vi "PyrometerSettings.vi"() -> ()   [LabVIEW 2018]
uses:
  C:/Users/bowenm/Git/Acquisition/Instruments/ImagingPyrometer/Kineses/ThorLabs.MotionControl.KCube.DCServoCLI.dll
  Kineses/ThorLabs.MotionControl.KCube.DCServoCLI.dll
  Global Variables.vi
  <vilib>/Utility/file.llb/Read Delimited Spreadsheet (string).vi
  C:/Users/bowenm/Git/Acquisition/Instruments/ImagingPyrometer/Kineses/Thorlabs.MotionControl.Controls.dll
  Kineses/Thorlabs.MotionControl.Controls.dll
  <instrlib>/Thorlabs_FW102C/Thorlabs_FW102C.lvlib
panel:
  in  "Set":bool
  out "Position Error":bool
  out "tdms file out":refnum<k34>
  out "RFW wls":string[](array[string])=["800", "900", "850", "750", "700", "600"]
  out "TFW wls":string[](array[string])=["1000", "850", "800", "700", "650", "600"]
  in  "Tab Control":enum32{"400-700nm", "700-1100nm"}(tab)
  in  "VisTFW Wavelength":u16(ring) caption="Wavelength 1" items=["600", "650", "700"]
  in  "VisRFW Wavelength":u16(ring) caption="Wavelength 2" items=["600", "700"]
  in  "NIRRFW Wavelengths":u16(ring) caption="Wavelength 2" items=["700", "750", "800", "850", "900"]
  in  "NIRTFW Wavelengths":u16(ring) caption="Wavelength 1" items=["700", "800", "850", "1000"]
  out "NDFs":dbl[](array[numeric])=[0.0, 20.0, 40.0, 60.0, 80.0, 100.0]
  in  "NeutralDensityFilter":u16(ring) items=["0", "20", "40", "60", "80", "100"]
  in  "NDFW Serial Port":string="COM17"
  out "NDFW102C out":i32
  out "RFW102C out":i32=1
  in  "RFW Serial Port":string="COM3"
  out "error out":errorcluster
  out "TFW102C out":i32
  in  "TFW Serial Port":string="COM4"
  out "MotorMoving":bool
  out "Device":refnum<k24>
  in  "stop":bool
  in  "KCubeDCServoControl":refnum<k24>(container)
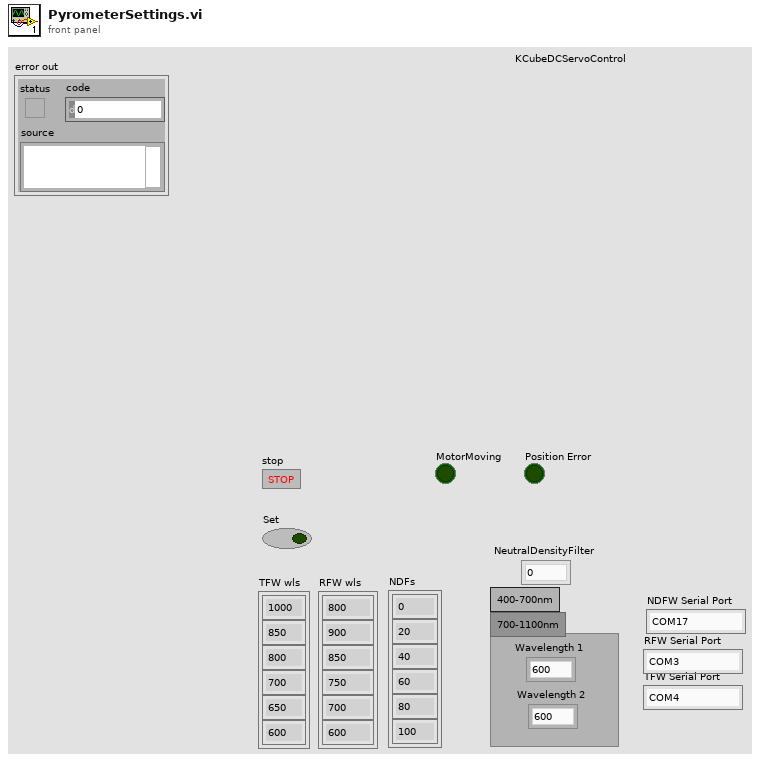
[diagram p1: front panel]
types:
  T1 = enum16{"open", "open or create", "create or replace", "create", "open (read-only)"}
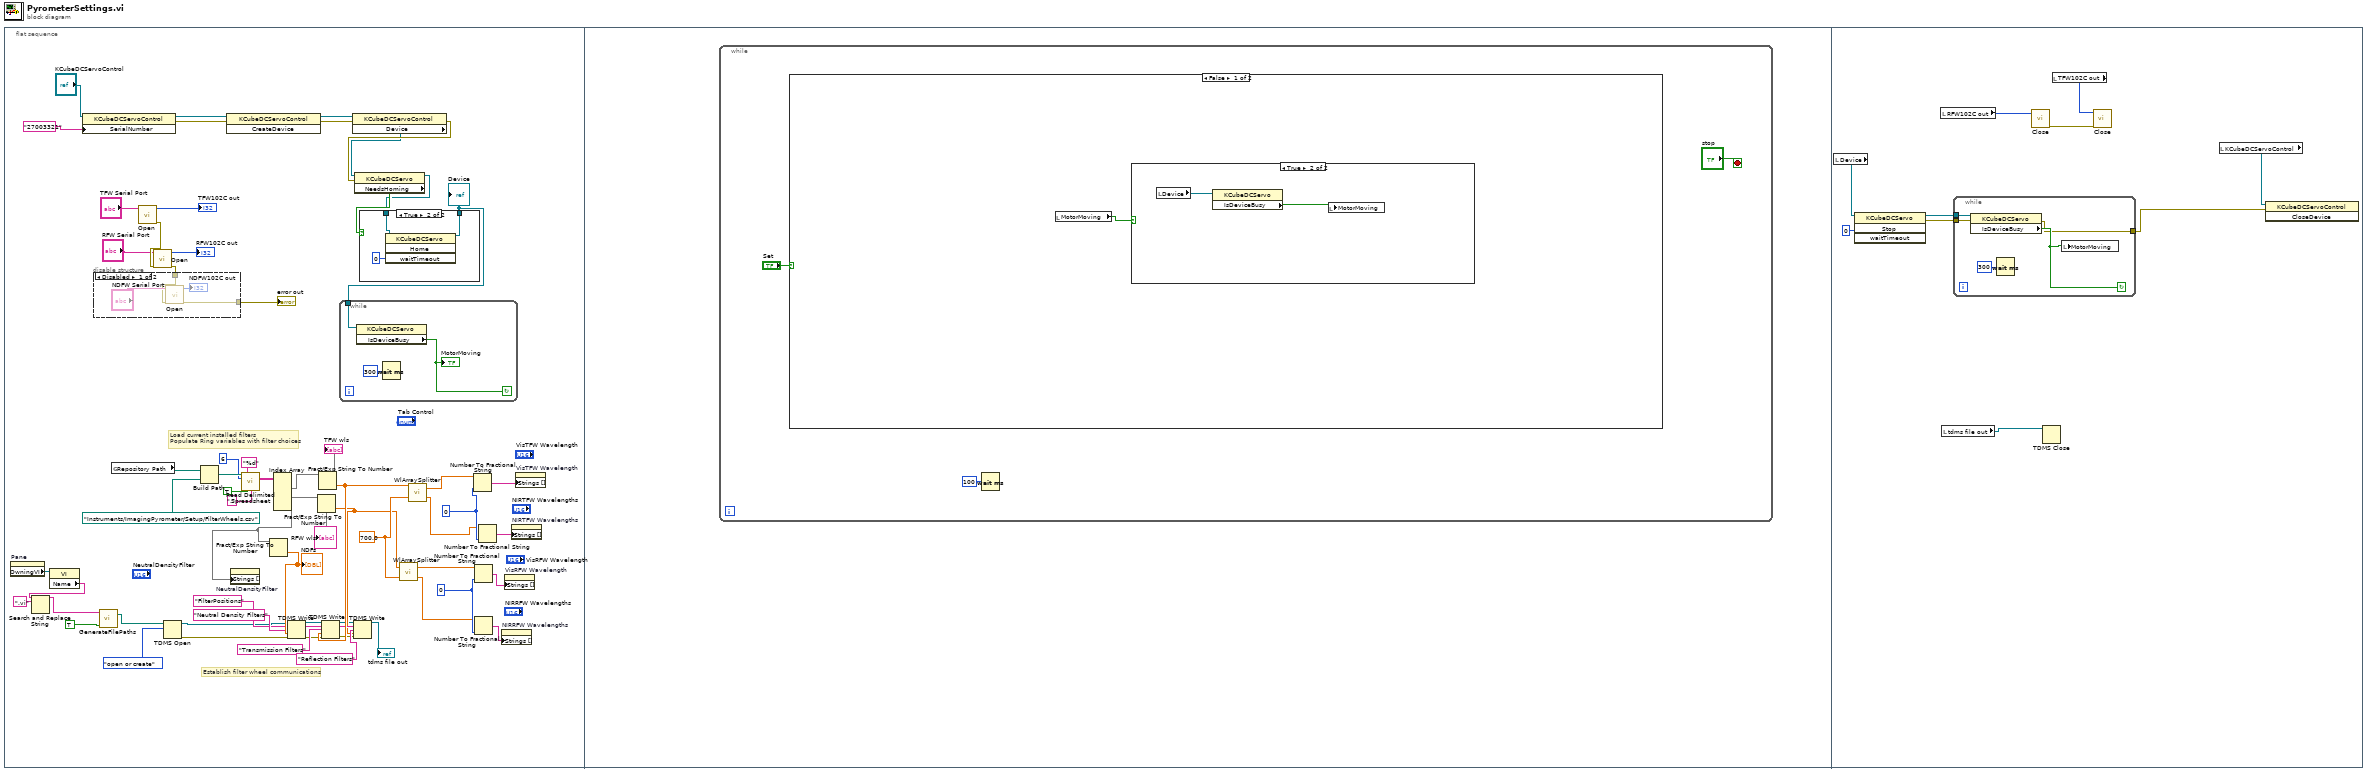
[diagram p0: block diagram]
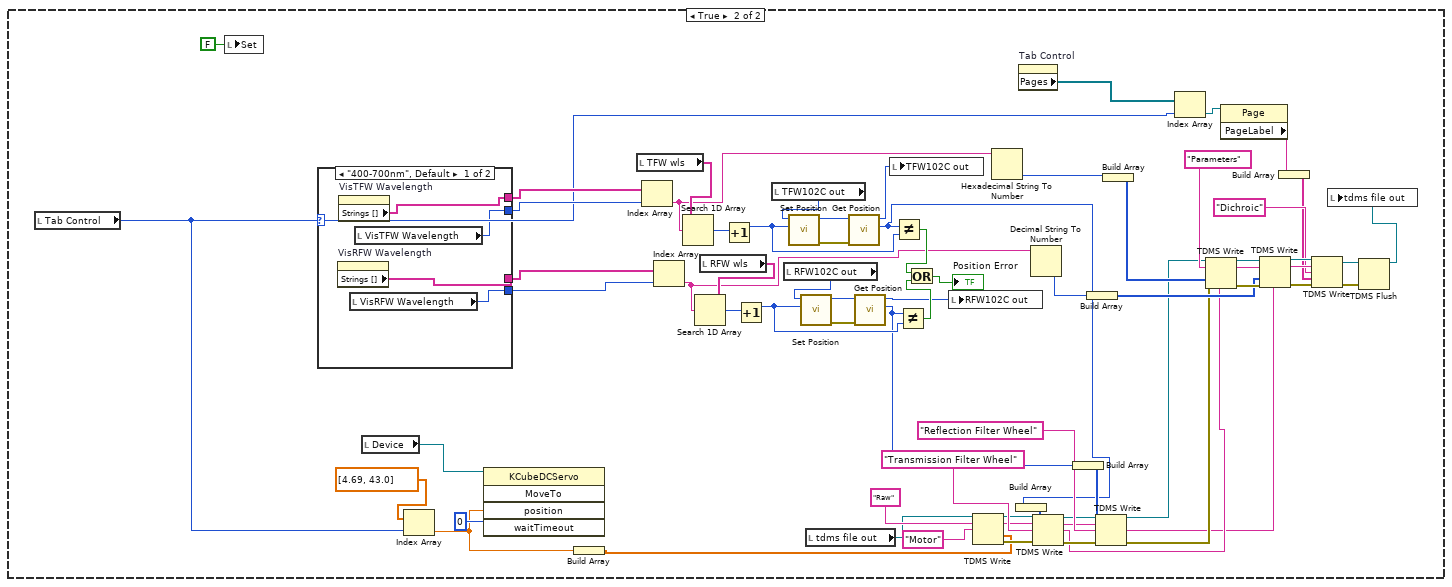
[diagram p5: hidden frame]
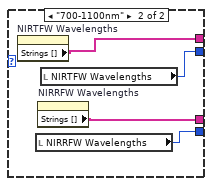
[diagram p6: hidden frame]
diagram:
  n1 = flat-sequence {
    frame #0 {
      w29 = i16 0 ("precision (6)")
      w30 = 700.0 ("Cutoff Wavelength")
      w39 = i16 0 ("precision (6)")
      # "Load current installed filters\nPopulate Ring variables with filter choices"
      # "Establish filter wheel communications"
      n2 = property on="Pane" class="Pane"() -> ("OwningVI"=w7:refnum<vi>)  [unwired: 2 in, 2 out]
      n3 = property class="VI"(reference=w7) -> ("Name"=w3:string)  [unwired: 1 in, 2 out]
      n4 = Search and Replace String(input string=w3, search string=".vi") -> (result string=w5:string)  [unwired: 6 in, 3 out]
      n5 = property class="KCubeDCServoControl"(reference="KCubeDCServoControl", "SerialNumber"="27003321") -> (reference out=w55:refnum<k24>, error out=w56:errorcluster)  [unwired: 1 in]
      n6 = call "GenerateFilePaths.vi"("Logfile? (F)"=TRUE ("Logfile?"), "Device Name"=w5) -> ("Path"=w2:path)  [unwired: 3 in]
      n7 = global read "Global Variables.vi" "Repository Path"() -> (w41:path)
      n8 = call <instrlib>:"Open.vi"("Serial Port"="TFW Serial Port") -> ("error out"=w50:errorcluster, "FW102C out"=→"TFW102C out":i32)  [unwired: 8 in, 1 out]
      n9 = call <instrlib>:"Open.vi"("error in (no error)"=w50, "Serial Port"="RFW Serial Port") -> ("error out"=w51:errorcluster, "FW102C out"=→"RFW102C out":i32)  [unwired: 7 in, 1 out]
      n10 = disable-structure shown="Disabled" {
        disable-tunnel: [w66 w68] -> w52
        disable-tunnel: w51 -> [w64 w68]
        frame Disabled {
          n11 = call <instrlib>:"Open.vi"("error in (no error)"=w64, "Serial Port"="NDFW Serial Port") -> ("error out"=w66:errorcluster, "FW102C out"=→"NDFW102C out":i32)  [unwired: 7 in, 1 out]
        }
        frame Enabled {
        }
      }
      "error out" <- w52
      n12 = TDMS Open(10:T1."open or create" ("operation (0:open)"), 11:w2) -> (0:w13:errorcluster, 3:w14:refnum<k34>)  [unwired: 5 in]
      n13 = Build Path(base path=w41, name or relative path=path "Instruments/ImagingPyrometer/Setup/FilterWheels.csv" ("vi path")) -> (appended path=w42:path)
      n14 = invoke class="KCubeDCServoControl" method="CreateDevice"(reference=w55, error in=w56) -> (reference out=w57:refnum<k24>, error out=w58:errorcluster)  [unwired: 1 in, 1 out]
      n15 = call-poly <vilib>:"Read Delimited Spreadsheet.vi"("file path (dialog if empty)"=w42, "format (%s)"="%d", "number of rows (all:-1)"=6, "transpose? (F)"=TRUE, "delimiter (\\t)"="," ("delimiter (\\t)")) -> ("all rows"=w34:string[][])  [unwired: 5 in, 5 out]
      n16 = Index Array(array=w34) -> (element #1=w32:string[], element #2=w31:string[], element #3=w24:string[])  [unwired: 6 in]
      "TFW wls" <- w32
      "RFW wls" <- w31
      n17 = property on="NeutralDensityFilter" class="Ring (strict)"("Strings []"=w24) -> ()  [unwired: 2 in, 2 out]
      n18 = Fract/Exp String To Number(string=w24) -> (number=w23:dbl[])  [unwired: 3 in, 1 out]
      "NDFs" <- w23
      n19 = TDMS Write(0:w14, 5:"FilterPositions" ("group name in (Untitled)"), 7:"Neutral Density Filters", 9:w23, 11:w13) -> (4:w12:refnum<k34>, 6:w20:string, 15:w11:errorcluster)  [unwired: 1 in, 1 out]
      n20 = Fract/Exp String To Number(string=w31) -> (number=w15:dbl[])  [unwired: 3 in, 1 out]
      n21 = Fract/Exp String To Number(string=w32) -> (number=w19:dbl[])  [unwired: 3 in, 1 out]
      n22 = TDMS Write(0:w12, 5:w20, 7:"Transmission Filters", 9:w19, 11:w11) -> (4:w9:refnum<k34>, 6:w17:string, 15:w10:errorcluster)  [unwired: 1 in, 1 out]
      n23 = property class="KCubeDCServoControl"(reference=w57, error in=w58) -> (error out=w60:errorcluster, "Device"=w59:refnum<k24>)  [unwired: 1 out]
      n24 = TDMS Write(0:w9, 5:w17, 7:"Reflection Filters", 9:w15, 11:w10) -> (4:→"tdms file out":refnum<k34>)  [unwired: 1 in, 3 out]
      n25 = property class="KCubeDCServo"(reference=w59, error in=w60) -> (reference out=w61:refnum<k24>, "NeedsHoming"=w62:bool)  [unwired: 1 out]
      n26 = case shown="True" w62 {
        tunnel: w61 -> [w72 w75]
        tunnel: [w72 w74] -> w63
        frame False {
        }
        frame True {
          n27 = invoke class="KCubeDCServo" method="Home"(reference=w75, "waitTimeout"=0) -> (reference out=w74:refnum<k24>)  [unwired: 2 in, 3 out]
        }
      }
      "Device" <- w63
      n28 = while {
        tunnel: w63 -> [w69]
        stop <- w71 continue-if-true
        n29 = property class="KCubeDCServo"(reference=w69) -> ("IsDeviceBusy"=w71:bool)  [unwired: 1 in, 2 out]
        "MotorMoving" <- w71
        n30 = Wait (ms)(milliseconds to wait=u32 300) -> ()  [unwired: 1 out]
      }
      n31 = call "WlArraySplitter.vi"("Cutoff Wavelength"=w30, "Wavelength Array"=w15) -> ("Higher Wavelengths"=w27:dbl[], "Lower Wavelengths"=w28:dbl[])
      n32 = call "WlArraySplitter.vi"("Cutoff Wavelength"=w30, "Wavelength Array"=w19) -> ("Higher Wavelengths"=w35:dbl[], "Lower Wavelengths"=w36:dbl[])
      n33 = Number To Fractional String(number=w36, precision (6)=w39) -> (F-format string=w38:string[])  [unwired: 2 in]
      n34 = Number To Fractional String(number=w28, precision (6)=w29) -> (F-format string=w25:string[])  [unwired: 2 in]
      n35 = Number To Fractional String(number=w27, precision (6)=w29) -> (F-format string=w26:string[])  [unwired: 2 in]
      n36 = Number To Fractional String(number=w35, precision (6)=w39) -> (F-format string=w37:string[])  [unwired: 2 in]
      n37 = property on="NIRRFW Wavelengths" class="Ring (strict)"("Strings []"=w26) -> ()  [unwired: 2 in, 2 out]
      n38 = property on="VisRFW Wavelength" class="Ring (strict)"("Strings []"=w25) -> ()  [unwired: 2 in, 2 out]
      n39 = property on="NIRTFW Wavelengths" class="Ring (strict)"("Strings []"=w37) -> ()  [unwired: 2 in, 2 out]
      n40 = property on="VisTFW Wavelength" class="Ring (strict)"("Strings []"=w38) -> ()  [unwired: 2 in, 2 out]
    }
    frame #1 {
      n41 = while {
        stop <- "stop" stop-if-true
        n42 = case shown="False" "Set" {
          frame False {
            n43 = local read "MotorMoving"() -> (w79:bool)
            n44 = case shown="True" w79 {
              frame False {
              }
              frame True {
                n45 = local read "Device"() -> (w80:refnum<k24>)
                n46 = property class="KCubeDCServo"(reference=w80) -> ("IsDeviceBusy"=w81:bool)  [unwired: 1 in, 2 out]
                n47 = local write "MotorMoving"(w81) -> ()
              }
            }
          }
          frame True {
            n48 = local read "Tab Control"() -> (w83:enum32{"400-700nm", "700-1100nm"})
            n49 = local write "Set"(FALSE ("Set")) -> ()
            n50 = case shown="\"400-700nm\", Default" w83 {
              tunnel: [w150 w154] -> w109
              tunnel: [w152 w157] -> w108
              tunnel: [w151 w155] -> w111
              tunnel: [w153 w156] -> w110
              frame "400-700nm", Default {
                n51 = property on="VisRFW Wavelength" class="Ring (strict)"() -> ("Strings []"=w150:string[])  [unwired: 2 in, 2 out]
                n52 = property on="VisTFW Wavelength" class="Ring (strict)"() -> ("Strings []"=w151:string[])  [unwired: 2 in, 2 out]
                n53 = local read "VisRFW Wavelength"() -> (w152:u16)
                n54 = local read "VisTFW Wavelength"() -> (w153:u16)
              }
              frame "700-1100nm" {
                n55 = property on="NIRTFW Wavelengths" class="Ring (strict)"() -> ("Strings []"=w155:string[])  [unwired: 2 in, 2 out]
                n56 = local read "NIRRFW Wavelengths"() -> (w157:u16)
                n57 = property on="NIRRFW Wavelengths" class="Ring (strict)"() -> ("Strings []"=w154:string[])  [unwired: 2 in, 2 out]
                n58 = local read "NIRTFW Wavelengths"() -> (w156:u16)
              }
            }
            n59 = local read "Device"() -> (w85:refnum<k24>)
            n60 = Index Array(array=dbl[] [4.69, 43.0], index=w83) -> (element=w86:dbl)
            n61 = invoke class="KCubeDCServo" method="MoveTo"(reference=w85, "position"=w86, "waitTimeout"=0) -> ()  [unwired: 2 in, 5 out]
            n62 = Build Array(w86) -> (w84:dbl[])
            n63 = local read "TFW wls"() -> (w136:string[])
            n64 = Index Array(array=w111, index=w110) -> (element=w132:string)
            n65 = Index Array(array=w109, index=w108) -> (element=w126:string)
            n66 = Search 1D Array(1D array=w136, element=w132) -> (index of element=w137:i32)  [unwired: 1 in]
            n67 = local read "RFW wls"() -> (w141:string[])
            n68 = Search 1D Array(1D array=w141, element=w126) -> (index of element=w140:i32)  [unwired: 1 in]
            n69 = Increment(x=w137) -> (x+1=w147:i32)
            n70 = Increment(x=w140) -> (x+1=w146:i32)
            n71 = local read "TFW102C out"() -> (w138:i32)
            n72 = local read "RFW102C out"() -> (w139:i32)
            n73 = call <instrlib>:"Set Position.vi"("Position"=w147, "FW102C in"=w138) -> ("error out"=w143:errorcluster, "FW102C out"=w142:i32)  [unwired: 8 in]
            n74 = call <instrlib>:"Set Position.vi"("Position"=w146, "FW102C in"=w139) -> ("error out"=w144:errorcluster, "FW102C out"=w145:i32)  [unwired: 8 in]
            n75 = local read "tdms file out"() -> (w95:refnum<k34>)
            n76 = call <instrlib>:"Get Position.vi"("error in (no error)"=w143, "FW102C in"=w142) -> ("Position"=w91:i32, "FW102C out"=w134:i32)  [unwired: 7 in, 1 out]
            n77 = call <instrlib>:"Get Position.vi"("error in (no error)"=w144, "FW102C in"=w145) -> ("Position"=w92:i32, "FW102C out"=w133:i32)  [unwired: 7 in, 1 out]
            n78 = local write "TFW102C out"(w134) -> ()
            n79 = Not Equal?(x=w91, y=w147) -> (x != y?=w148:bool)
            n80 = Not Equal?(x=w92, y=w146) -> (x != y?=w149:bool)
            n81 = Or(x=w148, y=w149) -> (x .or. y?=→"Position Error":bool)
            n82 = local write "RFW102C out"(w133) -> ()
            n83 = TDMS Write(0:w95, 5:"Raw", 7:"Motor", 9:w84) -> (4:w98:refnum<k34>, 6:w99:string, 15:w101:errorcluster)  [unwired: 2 in, 1 out]
            n84 = Hexadecimal String To Number(string=w132) -> (number=w131:u32)  [unwired: 2 in, 1 out]
            n85 = Build Array(w91) -> (w100:i32[])
            n86 = property on="Tab Control" class="TabCtl (strict)"() -> ("Pages"=w119:refnum<vi>[])  [unwired: 2 in, 2 out]
            n87 = Decimal String To Number(string=w126) -> (offset past number=w125:i32)  [unwired: 2 in, 1 out]
            n88 = TDMS Write(0:w98, 5:w99, 7:"Transmission Filter Wheel", 9:w100, 11:w101) -> (4:w104:refnum<k34>, 6:w102:string, 8:w90:string, 15:w105:errorcluster)  [unwired: 1 in]
            n89 = Build Array(w92) -> (w103:i32[])
            n90 = Build Array(w125) -> (w124:i32[])
            n91 = TDMS Write(0:w104, 5:w102, 7:"Reflection Filter Wheel", 9:w103, 11:w105) -> (4:w93:refnum<k34>, 8:w89:string, 15:w94:errorcluster)  [unwired: 1 in, 1 out]
            n92 = Build Array(w131) -> (w130:u32[])
            n93 = Index Array(array=w119, index=w83) -> (element=w118:refnum<vi>)
            n94 = TDMS Write(0:w93, 5:"Parameters", 7:w90, 9:w130, 11:w94) -> (4:w129:refnum<k34>, 6:w128:string, 15:w127:errorcluster)  [unwired: 1 in, 1 out]
            n95 = property class="Page"(reference=w118) -> ("PageLabel"=w117:string)  [unwired: 1 in, 2 out]
            n96 = TDMS Write(0:w129, 5:w128, 7:w89, 9:w124, 11:w127) -> (4:w123:refnum<k34>, 6:w122:string, 15:w121:errorcluster)  [unwired: 1 in, 1 out]
            n97 = Build Array(w117) -> (w116:string[])
            n98 = TDMS Write(0:w123, 5:w122, 7:"Dichroic", 9:w116, 11:w121) -> (4:w113:refnum<k34>, 15:w112:errorcluster)  [unwired: 1 in, 2 out]
            n99 = TDMS Flush(4:w112, 7:w113) -> (3:w114:refnum<k34>)  [unwired: 1 out]
            n100 = local write "tdms file out"(w114) -> ()
          }
        }
        n101 = Wait (ms)(milliseconds to wait=u32 100) -> ()  [unwired: 1 out]
      }
    }
    frame #2 {
      n102 = local read "Device"() -> (w167:refnum<k24>)
      n103 = invoke class="KCubeDCServo" method="Stop"(reference=w167, "waitTimeout"=0) -> (reference out=w164:refnum<k24>, error out=w165:errorcluster)  [unwired: 2 in, 2 out]
      n104 = local read "RFW102C out"() -> (w159:i32)
      n105 = local read "tdms file out"() -> (w158:refnum<k34>)
      n106 = while {
        tunnel: w164 -> [w172]
        tunnel: [w169] -> w166
        tunnel: w165 -> [w168]
        stop <- w170 continue-if-true
        n107 = property class="KCubeDCServo"(reference=w172, error in=w168) -> (error out=w169:errorcluster, "IsDeviceBusy"=w170:bool)  [unwired: 1 out]
        n108 = Wait (ms)(milliseconds to wait=u32 300) -> ()  [unwired: 1 out]
        n109 = local write "MotorMoving"(w170) -> ()
      }
      n110 = call <instrlib>:"Close.vi"("FW102C in"=w159) -> ("error out"=w161:errorcluster)  [unwired: 10 in]
      n111 = TDMS Close(11:w158) -> ()  [unwired: 1 in, 2 out]
      n112 = local read "TFW102C out"() -> (w160:i32)
      n113 = call <instrlib>:"Close.vi"("error in (no error)"=w161, "FW102C in"=w160) -> ()  [unwired: 9 in, 1 out]
      n114 = local read "KCubeDCServoControl"() -> (w163:refnum<k24>)
      n115 = invoke class="KCubeDCServoControl" method="CloseDevice"(reference=w163, error in=w166) -> ()  [unwired: 1 in, 3 out]
    }
  }
